vi "Read Camera Link Settings (SubVI).vi"(11 "Settings File Name":path=path "C:/MWT/Config.ini") -> (1 "Tap Configuration":string, 2 "Signal Mapping":string, 3 "CL Configuration":string)   [LabVIEW 2020]
uses:
  <vilib>/Utility/config.llb/Read Key (String).vi
  <vilib>/Utility/config.llb/Write Key (String).vi
  <vilib>/Utility/config.llb/NI_LVConfig.lvlib
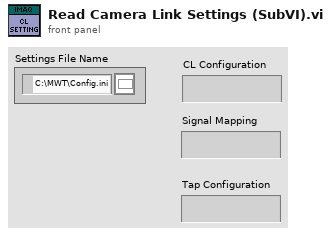
[diagram p1: front panel]
types:
  T1 = typedef "NI_LVConfig.lvlib/Config Data RefNum.ctl" = refnum<k1>
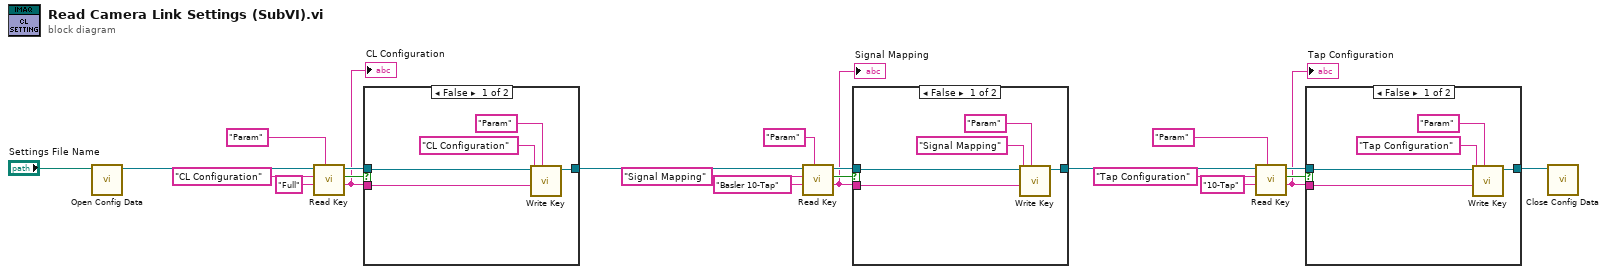
[diagram p0: block diagram]
diagram:
  n1 = call <vilib>:"Open Config Data.vi"("configuration file path"="Settings File Name") -> ("refnum"=w21:T1)  [unwired: 8 in, 2 out]
  n2 = call-poly <vilib>:"Read Key.vi"("section"="Param", "default value"="Full", "key"="CL Configuration" ("section"), "refnum"=w21) -> ("value"=w17:string, "found?"=w19:bool, "refnum out"=w18:T1)  [unwired: 4 in, 1 out]
  "CL Configuration" <- w17
  n3 = case shown="False" w19 {
    tunnel: w18 -> [w26 w29]
    tunnel: [w25 w29] -> w10
    tunnel: w17 -> [w24 _]
    frame False {
      n4 = call-poly <vilib>:"Write Key.vi"("section"="Param", "value"=w24, "key"="CL Configuration" ("section"), "refnum"=w26) -> ("refnum out"=w25:T1)  [unwired: 5 in, 2 out]
    }
    frame True {
    }
  }
  n5 = call-poly <vilib>:"Read Key.vi"("section"="Param", "default value"="Basler 10-Tap", "key"="Signal Mapping" ("section"), "refnum"=w10) -> ("value"=w1:string, "found?"=w13:bool, "refnum out"=w14:T1)  [unwired: 4 in, 1 out]
  "Signal Mapping" <- w1
  n6 = case shown="False" w13 {
    tunnel: w14 -> [w32 w35]
    tunnel: [w31 w35] -> w4
    tunnel: w1 -> [w30 _]
    frame False {
      n7 = call-poly <vilib>:"Write Key.vi"("section"="Param", "value"=w30, "key"="Signal Mapping" ("section"), "refnum"=w32) -> ("refnum out"=w31:T1)  [unwired: 5 in, 2 out]
    }
    frame True {
    }
  }
  n8 = call-poly <vilib>:"Read Key.vi"("section"="Param", "default value"="10-Tap", "key"="Tap Configuration" ("section"), "refnum"=w4) -> ("value"=w2:string, "found?"=w7:bool, "refnum out"=w6:T1)  [unwired: 4 in, 1 out]
  "Tap Configuration" <- w2
  n9 = case shown="False" w7 {
    tunnel: w6 -> [w38 w41]
    tunnel: [w37 w41] -> w3
    tunnel: w2 -> [w36 _]
    frame False {
      n10 = call-poly <vilib>:"Write Key.vi"("section"="Param", "value"=w36, "key"="Tap Configuration" ("section"), "refnum"=w38) -> ("refnum out"=w37:T1)  [unwired: 5 in, 2 out]
    }
    frame True {
    }
  }
  n11 = call <vilib>:"Close Config Data.vi"("refnum"=w3) -> ()  [unwired: 9 in, 2 out]
